vi "VCS Set Sensor Type.vi"(8 "error in (no error)":errorcluster, 9 "SensorType":u16(ring) items=["Unknown sensor", "Incremental encoder with index (3-channel)", "Incremental encoder without index (2-channel)", "Hall sensors", "SSI encoder binary coded", "SSI encoder grey coded"], 11 "axis in":cluster{"keyHandle":u32, "nodeId":u16}={"keyHandle"=0, "nodeId"=1}) -> (0 "error out":errorcluster, 3 "axis out":cluster{"keyHandle":u32, "nodeId":u16}={"keyHandle"=0, "nodeId"=1})   [LabVIEW 2018]
doc: "With function <B>VCS_SetSensorType</B> it is possible to write the sensor type."
uses:
  Resources/EposCmd.dll
  Resources/EposCmd64.dll
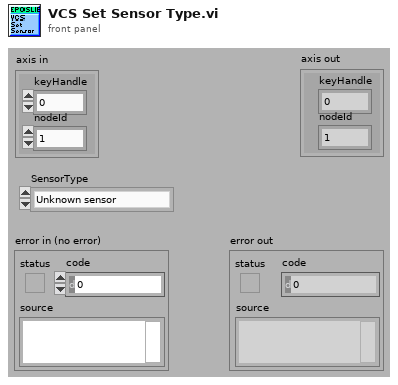
[diagram p1: front panel]
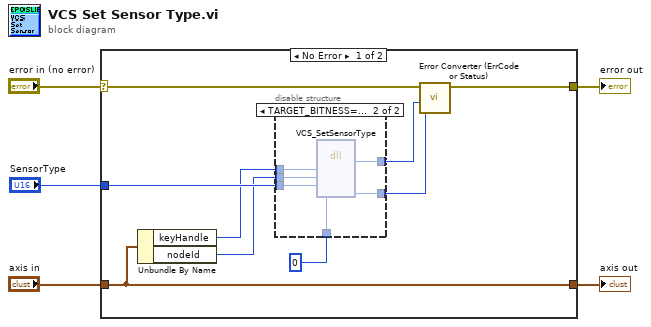
[diagram p0: block diagram]
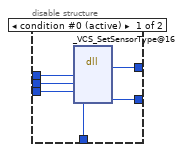
[diagram p2: hidden frame]
diagram:
  n1 = case shown="No Error" "error in (no error)" {
    selector: "error in (no error)" -> [w12 w27]
    tunnel: "axis in" -> [w14 w28]
    tunnel: [w14 w28] -> w4
    tunnel: [w13 w27] -> w3
    tunnel: "SensorType" -> [w11 _]
    frame No Error {
      n2 = Unbundle By Name(w14) -> ("keyHandle"=w10:u32, "nodeId"=w9:u16)
      n3 = disable-structure shown="TARGET_BITNESS==64" {
        disable-tunnel: w11 -> [w20 w26]
        disable-tunnel: w10 -> [w19 w25]
        disable-tunnel: w9 -> [w18 w24]
        disable-tunnel: u32 0 ("pErrorCode") -> [w17 w23]
        disable-tunnel: [w16 w22] -> w7
        disable-tunnel: [w15 w21] -> w6
        frame condition #0 (active) {
          n4 = dll-call lib="C:/Projeto em LabVIEW/EPOS-LabVIEW-Instrument-Driver-En/LabVIEW/maxon EPOS/Resources/EposCmd.*" fn="_VCS_SetSensorType@16"("KeyHandle"=w19, "NodeId"=w18, "SensorType"=w20, "pErrorCode"=w17) -> (w15:i32, "pErrorCode"=w16:u32)  [unwired: 6 in, 2 out]
        }
        frame condition #1 {
          n5 = dll-call lib="C:/setup/Resources/EposCmd64.*" fn="VCS_SetSensorType" ("EposCmd.dll:_VCS_SetSensorType@16")("KeyHandle"=w25, "NodeId"=w24, "SensorType"=w26, "pErrorCode"=w23) -> ("Rückgabetyp"=w21:i32, "pErrorCode"=w22:u32)  [unwired: 6 in, 2 out]
        }
      }
      n6 = call "Error Converter (ErrCode or Status).vi"("error code"=w7, "return type"=w6, "error in (no error)"=w12) -> ("error out"=w13:errorcluster)  [unwired: 7 in]
    }
    frame Error {
    }
  }
  "error out" <- w3
  "axis out" <- w4
